vi "Query Available Printers.vi"(8 "error in (no error)":errorcluster) -> (0 "error out":errorcluster, 2 "default printer":string, 3 "system configured printers":string[](array[string]))   [LabVIEW 2017, in "NI_ReportGenerationCore.lvlib"]
doc: "Lists the printers available on the computer, including the default printer in LabVIEW."
uses:
  <vilib>/Utility/NIReport.llb/NI_ReportGenerationCore.lvlib
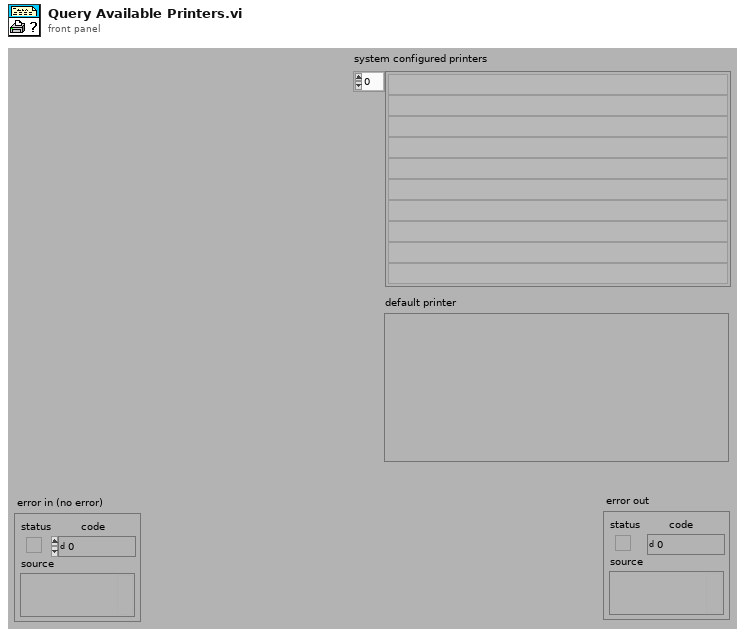
[diagram p1: front panel]
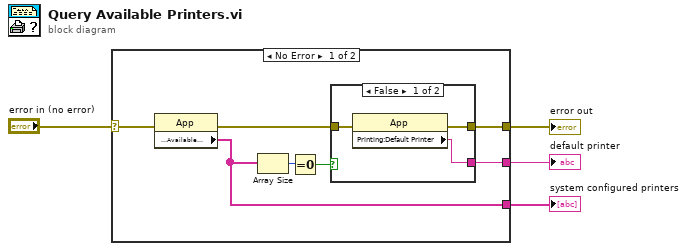
[diagram p0: block diagram]
diagram:
  n1 = case shown="No Error" "error in (no error)" {
    selector: "error in (no error)" -> [w11 w16]
    tunnel: [w7 w16] -> w3
    tunnel: [w6 _] -> w2
    tunnel: [w5 _] -> w1
    frame No Error {
      n2 = property class="App"(error in=w11) -> (error out=w8:errorcluster, "Printing:Available Printers"=w5:string[])  [unwired: 1 in, 1 out]
      n3 = Array Size(array=w5) -> (size(s)=w10:i32)
      n4 = Equal To 0?(x=w10) -> (x = 0?=w9:bool)
      n5 = case shown="False" w9 {
        tunnel: [w14 _] -> w6
        tunnel: w8 -> [w13 w15]
        tunnel: [w12 w15] -> w7
        frame False {
          n6 = property class="App"(error in=w13) -> (error out=w12:errorcluster, "Printing:Default Printer"=w14:string)  [unwired: 1 in, 1 out]
        }
        frame True {
        }
      }
    }
    frame Error {
    }
  }
  "error out" <- w3
  "default printer" <- w2
  "system configured printers" <- w1
